vi "Pointer.In-Place Read (String).vi"(8 "error in (no error)":errorcluster, 10 "allocated string in":string, 11 "pointer in":u64) -> (0 "error out":errorcluster, 2 "string out":string, 3 "pointer out":u64)   [LabVIEW 2016, in "VeriStand Data.lvlib"]
doc: "Reads a number of values, specified by the size of the provided <B>array</B>, from the provided <B>pointer</B>."
uses:
  VeriStand Data.lvlib
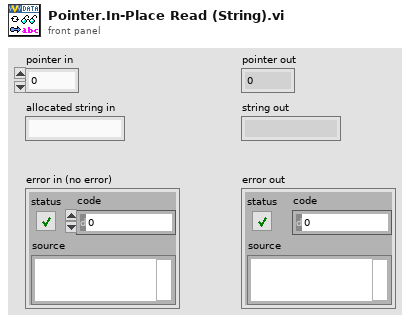
[diagram p1: front panel]
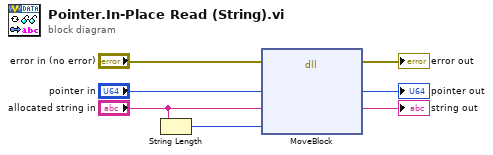
[diagram p0: block diagram]
diagram:
  n1 = String Length(string="allocated string in") -> (length=w1:i32)
  n2 = dll-call lib="LabVIEW" fn="MoveBlock"(error in="error in (no error)", "ps"="pointer in", "pd"="allocated string in", "size"=w1) -> (error out=→"error out":errorcluster, "ps"=→"pointer out":u64, "pd"=→"string out":string)  [unwired: 4 in, 1 out]
